vi "TCL Select Fragments NfragsNcriteria.vi"(0 "event file":path, 1 "fragments":string[](array[string]), 3 "primary key":string, 4 "criteria":T1(array[cluster]), 5 "error in (no error)":errorcluster) -> (6 "fragments out":string[](array[string]), 7 "matches":string[][](array[string]), 8 "error out":errorcluster)   [LabVIEW 2010]
uses:
  <vilib>/Utility/file.llb/Read From Spreadsheet File (string).vi
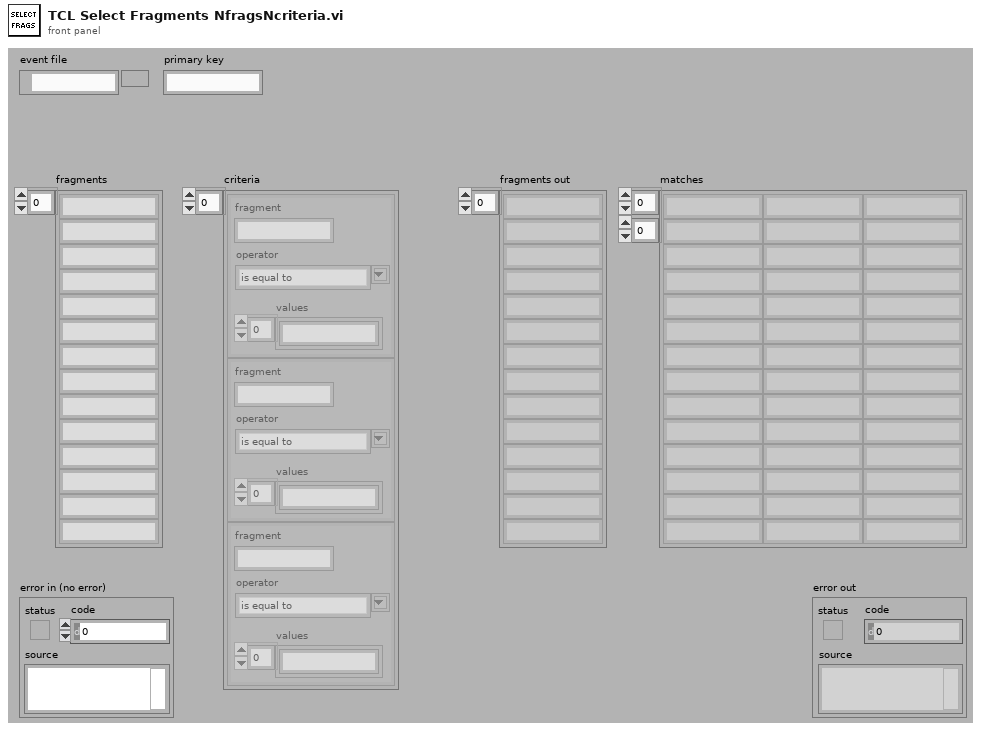
[diagram p1: front panel]
types:
  T1 = cluster{"fragment":string, "values":string[], "operator":string}[]
  T2 = cluster{"fragment":string, "values":string[], "operator":string}
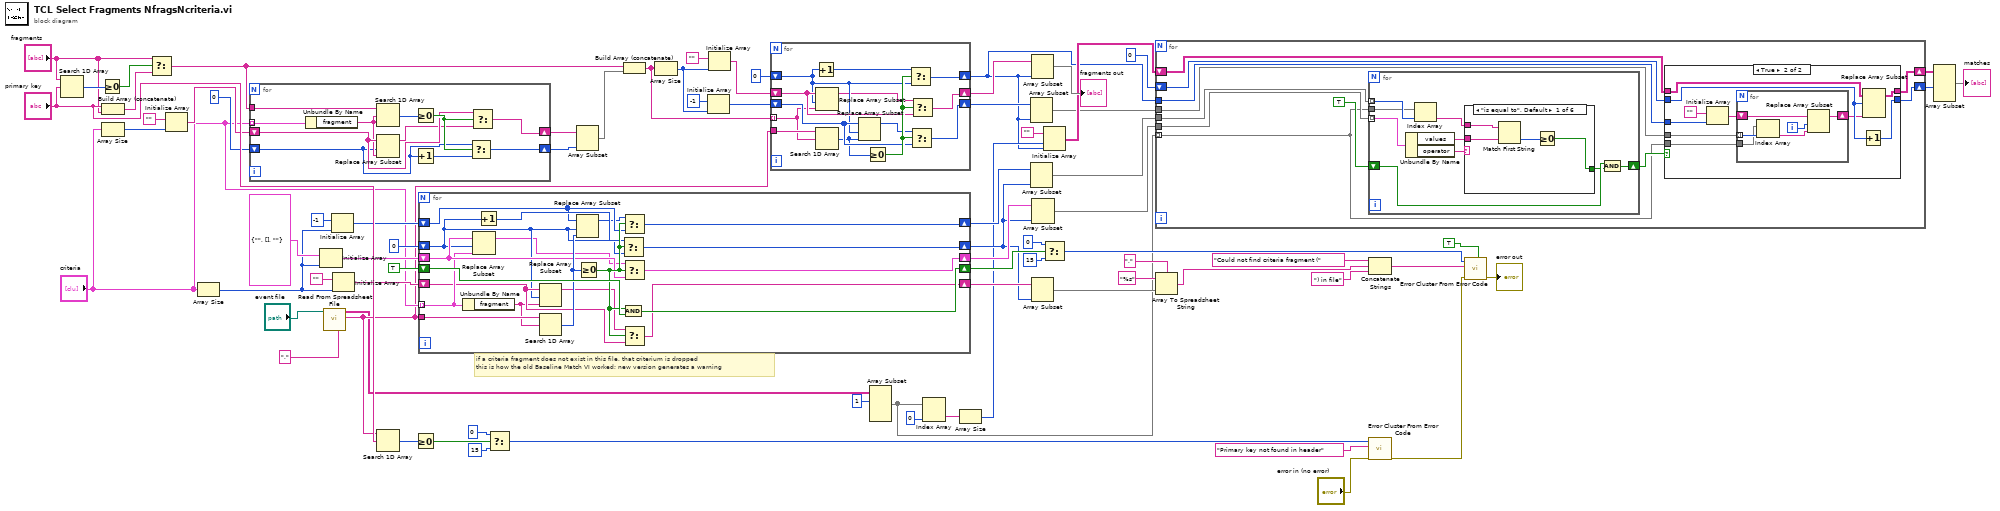
[diagram p0: block diagram]
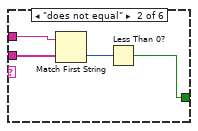
[diagram p3: hidden frame]
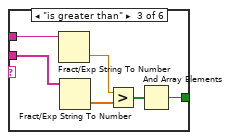
[diagram p4: hidden frame]
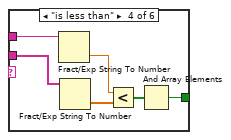
[diagram p5: hidden frame]
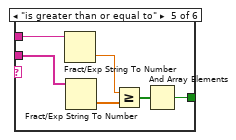
[diagram p6: hidden frame]
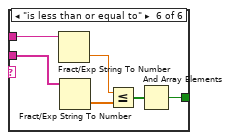
[diagram p7: hidden frame]
diagram:
  # "if a criteria fragment does not exist in this file, that criterium is dropped\nthis is how the old Baseline Match VI worked; new version generates a warning"
  n1 = Search 1D Array(1D array="fragments", element="primary key") -> (index of element=w76:i32)  [unwired: 1 in]
  n2 = Greater Or Equal To 0?(x=w76) -> (x >= 0?=w75:bool)
  n3 = Build Array (concatenate)("primary key", "fragments") -> (w74:string[])
  n4 = Array Size(array="criteria") -> (size(s)=w64:i32)
  n5 = Select(t="fragments", s=w75, f=w74) -> (s? t:f=w62:string[])
  n6 = Initialize Array("", w64) -> (w65:string[])
  n7 = Array Size(array="criteria") -> (size(s)=w51:i32)
  n8 = for {
    shift-right: [w87] -> w61
    shift-left: w65 -> [w82]
    tunnel: "criteria" -> [w85] mode=indexing
    shift-right: [w88] -> w60
    shift-left: 0 -> [w78]
    tunnel: w62 -> [w86]
    n9 = Unbundle By Name(w85) -> ("fragment"=w81:string)
    n10 = Search 1D Array(1D array=w86, element=w81) -> (index of element=w84:i32)  [unwired: 1 in]
    n11 = Replace Array Subset(array=w82, new element=w81, index=w78) -> (w80:string[])
    n12 = Greater Or Equal To 0?(x=w84) -> (x >= 0?=w83:bool)
    n13 = Increment(x=w78) -> (x+1=w79:i32)
    n14 = Select(t=w78, s=w83, f=w79) -> (s? t:f=w88:i32)
    n15 = Select(t=w82, s=w83, f=w80) -> (s? t:f=w87:string[])
  }
  n16 = Initialize Array(T2 {"fragment"="", "values"=[], "operator"=""}, w51) -> (w54:T1)
  n17 = call-poly <vilib>:"Read From Spreadsheet File.vi"("delimiter (\\t)"="," ("delimiter (\\t)"), "file path (dialog if empty)"="event file") -> ("first row"=w24:string[], "all rows"=w21:string[][])  [unwired: 5 in, 3 out]
  n18 = Initialize Array(-1, w51) -> (w52:i32[])
  n19 = Initialize Array("", w51) -> (w57:string[])
  n20 = Search 1D Array(1D array=w24, element="primary key") -> (index of element=w72:i32)  [unwired: 1 in]
  n21 = Greater Or Equal To 0?(x=w72) -> (x >= 0?=w71:bool)
  n22 = for {
    shift-right: [w92] -> w43
    shift-left: w57 -> [w97]
    shift-right: [w106] -> w44
    shift-left: TRUE -> [w105]
    shift-right: [w93] -> w34
    shift-left: w54 -> [w99]
    shift-right: [w94] -> w32
    shift-left: w52 -> [w101]
    shift-right: [w102] -> w33
    shift-left: 0 -> [w96]
    tunnel: "criteria" -> [w98] mode=indexing
    tunnel: w24 -> [w107]
    n23 = Unbundle By Name(w98) -> ("fragment"=w95:string)
    n24 = Replace Array Subset(array=w99, new element=w98, index=w96) -> (w90:T1)
    n25 = Increment(x=w96) -> (x+1=w103:i32)
    n26 = Replace Array Subset(array=w97, new element=w95, index=w96) -> (w89:string[])
    n27 = Search 1D Array(1D array=w107, element=w95) -> (index of element=w100:i32)  [unwired: 1 in]
    n28 = Replace Array Subset(array=w101, new element=w100, index=w96) -> (w91:i32[])
    n29 = Greater Or Equal To 0?(x=w100) -> (x >= 0?=w104:bool)
    n30 = Select(t=w103, s=w104, f=w96) -> (s? t:f=w102:i32)
    n31 = And(x=w104, y=w105) -> (x .and. y?=w106:bool)
    n32 = Select(t=w91, s=w104, f=w101) -> (s? t:f=w94:i32[])
    n33 = Select(t=w90, s=w104, f=w99) -> (s? t:f=w93:T1)
    n34 = Select(t=w89, s=w104, f=w97) -> (s? t:f=w92:string[])
  }
  n35 = Select(t=0, s=w71, f=15) -> (s? t:f=w70:i32)
  n36 = Array Subset(array=w61, length=w60) -> (w59:string[])  [unwired: 1 in]
  n37 = Build Array (concatenate)(w62, w59) -> (w25:string[])
  n38 = Array Size(array=w25) -> (size(s)=w28:i32)
  n39 = Initialize Array(-1, w28) -> (w29:i32[])
  n40 = Initialize Array("", w28) -> (w26:string[])
  n41 = for {
    shift-right: [w113] -> w9
    shift-left: 0 -> [w115]
    shift-right: [w112] -> w22
    shift-left: w29 -> [w118]
    shift-right: [w111] -> w23
    shift-left: w26 -> [w116]
    tunnel: w25 -> [w108] mode=indexing
    tunnel: w24 -> [w114]
    n42 = Increment(x=w115) -> (x+1=w119:i32)
    n43 = Replace Array Subset(array=w116, new element=w108, index=w115) -> (w109:string[])
    n44 = Search 1D Array(1D array=w114, element=w108) -> (index of element=w117:i32)  [unwired: 1 in]
    n45 = Replace Array Subset(array=w118, new element=w117, index=w115) -> (w110:i32[])
    n46 = Greater Or Equal To 0?(x=w117) -> (x >= 0?=w120:bool)
    n47 = Select(t=w119, s=w120, f=w115) -> (s? t:f=w113:i32)
    n48 = Select(t=w110, s=w120, f=w118) -> (s? t:f=w112:i32[])
    n49 = Select(t=w109, s=w120, f=w116) -> (s? t:f=w111:string[])
  }
  n50 = Array Subset(array=w21, index (row)=1 ("index")) -> (w15:string[][])  [unwired: 3 in]
  n51 = Index Array(array=w15, index (col)=0 ("disabled index (col)")) -> (element=w13:string[])  [unwired: 1 in]
  n52 = Array Size(array=w13) -> (size(s)=w12:i32)
  n53 = Array Subset(array=w22, length=w9) -> (w8:i32[])  [unwired: 1 in]
  n54 = Array Subset(array=w32, length=w33) -> (w19:i32[])  [unwired: 1 in]
  n55 = Array Subset(array=w23, length=w9) -> (→"fragments out":string[])  [unwired: 1 in]
  n56 = Array Subset(array=w43, length=w33) -> (w42:string[])  [unwired: 1 in]
  n57 = Array Subset(array=w34, length=w33) -> (w18:T1)  [unwired: 1 in]
  n58 = Initialize Array("", w12, w9) -> (w11:string[][])
  n59 = Select(t=0, s=w44, f=15) -> (s? t:f=w47:i32)
  n60 = for {
    tunnel: w15 -> [w121] mode=indexing
    tunnel: w19 -> [w131]
    tunnel: w18 -> [w130]
    shift-right: [w126] -> w7
    shift-left: w11 -> [w127]
    shift-right: [w124] -> w2
    shift-left: 0 -> [w125]
    tunnel: w9 -> [w123]
    tunnel: w8 -> [w122]
    n61 = for {
      tunnel: w131 -> [w152] mode=indexing
      tunnel: w130 -> [w158] mode=indexing
      shift-right: [w156] -> w128
      shift-left: TRUE -> [w155]
      tunnel: w121 -> [w151]
      n62 = Unbundle By Name(w158) -> ("values"=w153:string[], "operator"=w157:string)
      n63 = Index Array(array=w151, index=w152) -> (element=w150:string)
      n64 = case shown="\"is equal to\", Default" w157 {
        tunnel: [w159 w163 w167 w173 w180 w186] -> w154
        tunnel: w153 -> [w162 w166 w171 w177 w183 w189]
        tunnel: w150 -> [w161 w165 w172 w178 w184 w190]
        frame "is equal to", Default {
          n65 = Match First String(2:w162, 3:w161) -> (0:w160:i32)  [unwired: 1 out]
          n66 = Greater Or Equal To 0?(x=w160) -> (x >= 0?=w159:bool)
        }
        frame "does not equal" {
          n67 = Match First String(2:w166, 3:w165) -> (0:w164:i32)  [unwired: 1 out]
          n68 = Less Than 0?(x=w164) -> (x < 0?=w163:bool)
        }
        frame "is greater than" {
          n69 = Fract/Exp String To Number(string=w172) -> (number=w169:dbl)  [unwired: 3 in, 1 out]
          n70 = Fract/Exp String To Number(string=w171) -> (number=w170:dbl[])  [unwired: 3 in, 1 out]
          n71 = Greater?(x=w169, y=w170) -> (0:w168:bool[])
          n72 = And Array Elements(Boolean array=w168) -> (logical AND=w167:bool)
        }
        frame "is less than" {
          n73 = Fract/Exp String To Number(string=w178) -> (number=w175:dbl)  [unwired: 3 in, 1 out]
          n74 = Fract/Exp String To Number(string=w177) -> (number=w176:dbl[])  [unwired: 3 in, 1 out]
          n75 = Less?(x=w175, y=w176) -> (x < y?=w174:bool[])
          n76 = And Array Elements(Boolean array=w174) -> (logical AND=w173:bool)
        }
        frame "is greater than or equal to" {
          n77 = Fract/Exp String To Number(string=w184) -> (number=w179:dbl)  [unwired: 3 in, 1 out]
          n78 = Fract/Exp String To Number(string=w183) -> (number=w182:dbl[])  [unwired: 3 in, 1 out]
          n79 = Greater Or Equal?(x=w179, y=w182) -> (x >= y?=w181:bool[])
          n80 = And Array Elements(Boolean array=w181) -> (logical AND=w180:bool)
        }
        frame "is less than or equal to" {
          n81 = Fract/Exp String To Number(string=w190) -> (number=w185:dbl)  [unwired: 3 in, 1 out]
          n82 = Fract/Exp String To Number(string=w189) -> (number=w188:dbl[])  [unwired: 3 in, 1 out]
          n83 = Less Or Equal?(x=w185, y=w188) -> (x <= y?=w187:bool[])
          n84 = And Array Elements(Boolean array=w187) -> (logical AND=w186:bool)
        }
      }
      n85 = And(x=w155, y=w154) -> (x .and. y?=w156:bool)
    }
    n86 = case shown="True" w128 {
      tunnel: w127 -> [w133 w137]
      tunnel: [w133 w134] -> w126
      tunnel: w125 -> [w132 w136]
      tunnel: [w132 w138] -> w124
      tunnel: w123 -> [_ w142]
      tunnel: w122 -> [_ w140]
      tunnel: w121 -> [_ w139]
      frame False {
      }
      frame True {
        n87 = Initialize Array("", w142) -> (w141:string[])
        n88 = for {
          shift-right: [w144] -> w135
          shift-left: w141 -> [w149]
          tunnel: w140 -> [w147] mode=indexing
          tunnel: w139 -> [w146]
          i -> [w148]
          n89 = Index Array(array=w146, index=w147) -> (element=w145:string)
          n90 = Replace Array Subset(array=w149, new element=w145, index=w148) -> (w144:string[])
        }
        n91 = Increment(x=w136) -> (x+1=w138:i32)
        n92 = Replace Array Subset(array=w137, new element=w135, index (row)=w136) -> (w134:string[][])  [unwired: 1 in]
      }
    }
  }
  n93 = Array To Spreadsheet String(delimiter (Tab)=",", array=w42, 3:"%s" ("format string")) -> (spreadsheet string=w38:string)
  n94 = Concatenate Strings("Could not find criteria fragment (" ("string"), w38, ") in file" ("string")) -> (w36:string)
  n95 = call <vilib>:"Error Cluster From Error Code.vi"("error in (no error)"="error in (no error)", "error message (\"\")"="Primary key not found in header" ("error message (\"\")"), "error code (0)"=w70) -> ("error out"=w48:errorcluster)  [unwired: 6 in]
  n96 = call <vilib>:"Error Cluster From Error Code.vi"("is warning? (False)"=TRUE, "error in (no error)"=w48, "error message (\"\")"=w36, "error code (0)"=w47) -> ("error out"=→"error out":errorcluster)  [unwired: 5 in]
  n97 = Array Subset(array=w7, length (row)=w2) -> (→"matches":string[][])  [unwired: 3 in]
